vi "Get EPTx Config Files.vi"(1 "password":string, 2 "IP_Address":string="0.0.0.0", 5 "username":string) -> (7 "EPTx Files":string[](array[string]))   [LabVIEW 2015]
uses:
  <vilib>/WebDAVClient/NI_WebDAV.lvlib
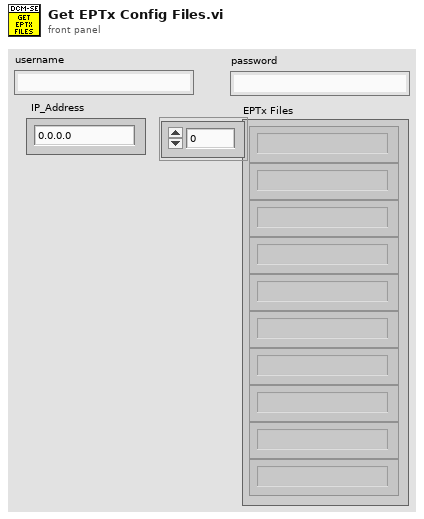
[diagram p1: front panel]
types:
  T1 = typedef "NI_WebDAV.lvlib/SessionHandle.ctl" = refnum<k1>
  T2 = typedef "NI_WebDAV.lvlib/FileInfo.ctl" = cluster{"type":string, "size":u64, "last modification":timestamp, "display name":string, "uri":string}
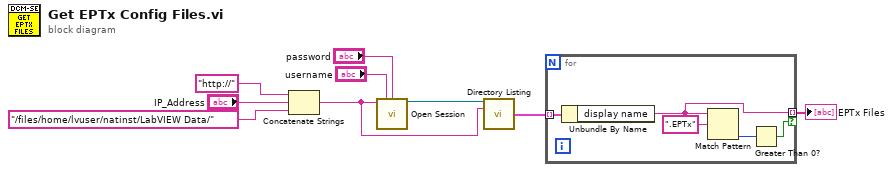
[diagram p0: block diagram]
diagram:
  n1 = Concatenate Strings("http://" ("host uri prefix"), "IP_Address", "/files/home/lvuser/natinst/LabVIEW Data/" ("string")) -> (w5:string)
  n2 = call <vilib>:"Open Session.vi"("host uri prefix"=w5, "username"="username", "password"="password") -> ("session handle out"=w6:T1)  [unwired: 11 in, 1 out]
  n3 = call <vilib>:"Directory Listing.vi"("session handle"=w6, "relative uri"=w5) -> ("file list"=w4:T2[])  [unwired: 10 in, 3 out]
  n4 = for {
    tunnel: w4 -> [w14] mode=indexing
    tunnel: [w10] -> w3 mode=indexing if=w11
    n5 = Unbundle By Name(w14) -> ("display name"=w10:string)
    n6 = Match Pattern(string=w10, regular expression=".EPTx") -> (offset past match=w12:i32)  [unwired: 1 in, 3 out]
    n7 = Greater Than 0?(x=w12) -> (x > 0?=w11:bool)
  }
  "EPTx Files" <- w3
